vi "dialog edit search paths.vi"(8 "error in":errorcluster, 11 "Plugin Search Paths":path[](array[path])) -> (0 "error out":errorcluster, 2 "Cancelled?":bool, 3 "Plugin Search Paths":path[](array[path]))   [LabVIEW 2013, in "configuration library.lvlib"]
uses:
  configuration library.lvlib
panel:
  in  "add":bool
  in  "remove":bool
  in  "Search Paths":i32(listbox)
  in  "Cancel":bool
  in  "OK":bool
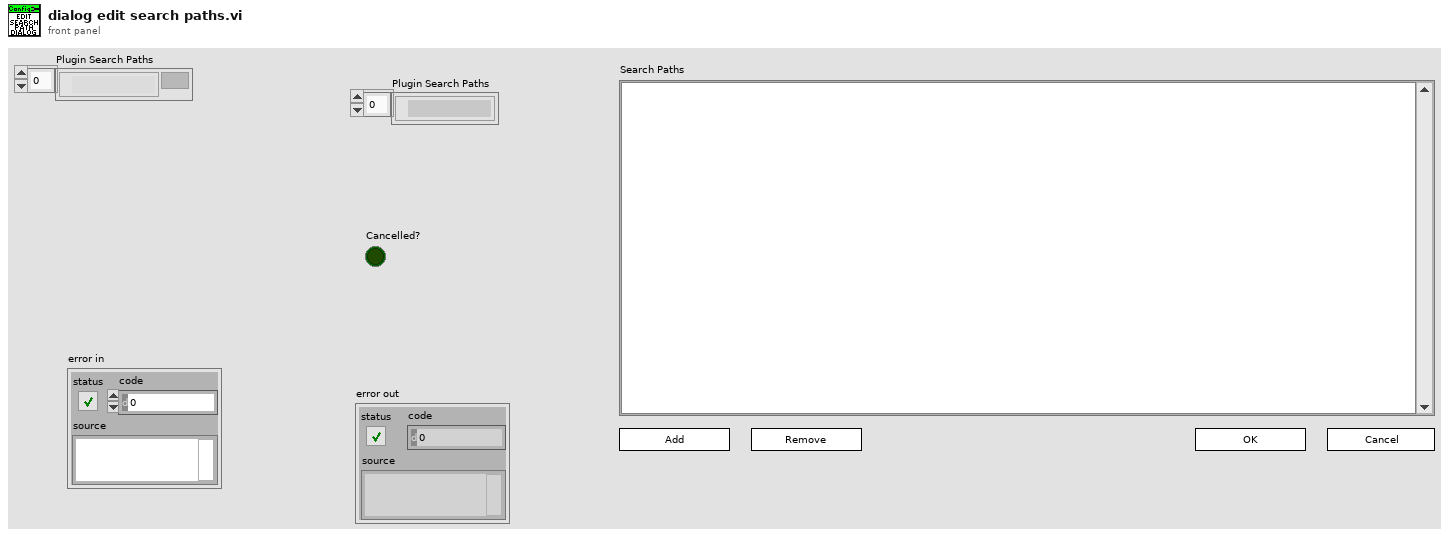
[diagram p1: front panel]
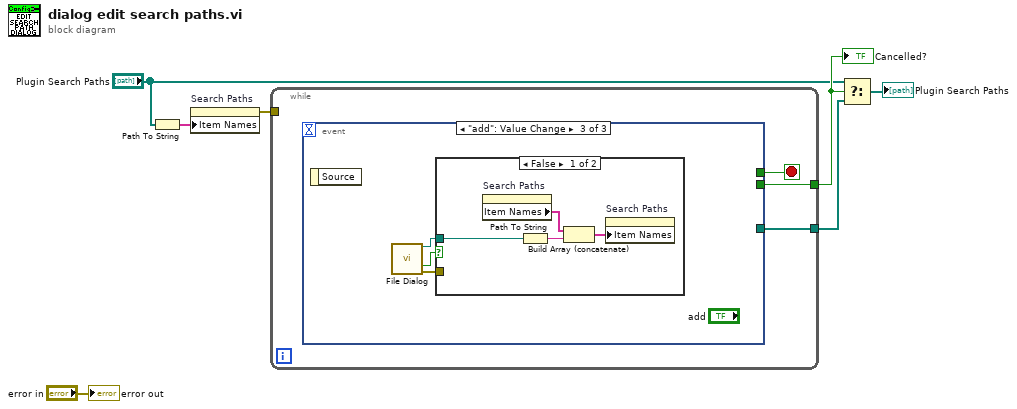
[diagram p0: block diagram]
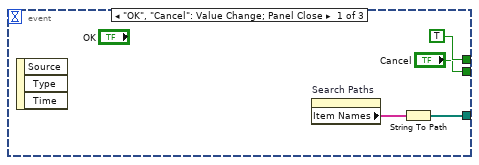
[diagram p2: hidden frame]
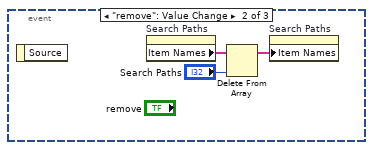
[diagram p3: hidden frame]
diagram:
  n1 = Path To String(path="Plugin Search Paths") -> (string=w2:string[])
  n2 = property on="Search Paths" class="LstBox (strict)"("Item Names"=w2) -> (error out=w1:errorcluster)  [unwired: 2 in, 1 out]
  n3 = while {
    tunnel: [w9] -> w5
    tunnel: [w8] -> w6
    tunnel: w1 -> [_]
    stop <- w10 stop-if-true
    n4 = event shown="[2] \"add\": Value Change" {
      selector: _ -> [_ _ _]
      dyn-events: _ -> [_ _ _]
      timeout: _ -> [_ _ _]
      tunnel: [TRUE _ _] -> w10
      tunnel: ["Cancel" _ _] -> w9
      tunnel: [w11 _ _] -> w8
      event "OK", "Cancel": Value Change; Panel Close {
        n5 = event-data() -> ()  [unwired: 1 in, 3 out]
        n6 = property on="Search Paths" class="LstBox (strict)"() -> ("Item Names"=w12:string[])  [unwired: 2 in, 2 out]
        n7 = String To Path(string=w12) -> (path=w11:path[])
      }
      event "remove": Value Change {
        n8 = event-data() -> ()  [unwired: 1 in, 1 out]
        n9 = property on="Search Paths" class="LstBox (strict)"() -> ("Item Names"=w17:string[])  [unwired: 2 in, 2 out]
        n10 = Delete From Array(array=w17, index="Search Paths") -> (array with subset deleted=w16:string[])  [unwired: 1 in, 1 out]
        n11 = property on="Search Paths" class="LstBox (strict)"("Item Names"=w16) -> ()  [unwired: 2 in, 2 out]
      }
      event "add": Value Change {
        n12 = event-data() -> ()  [unwired: 1 in, 1 out]
        n13 = call "File Dialog"() -> ("selected path"=w18:path, "cancelled"=w20:bool, "error out"=w19:errorcluster)  [unwired: 12 in, 1 out]
        n14 = case shown="False" w20 {
          tunnel: w19 -> [_ _]
          tunnel: w18 -> [w21 _]
          frame False {
            n15 = property on="Search Paths" class="LstBox (strict)"() -> ("Item Names"=w22:string[])  [unwired: 2 in, 2 out]
            n16 = Path To String(path=w21) -> (string=w24:string)
            n17 = Build Array (concatenate)(w22, w24) -> (w23:string[])
            n18 = property on="Search Paths" class="LstBox (strict)"("Item Names"=w23) -> ()  [unwired: 2 in, 2 out]
          }
          frame True {
          }
        }
      }
    }
  }
  "Cancelled?" <- w5
  n19 = Select(t="Plugin Search Paths", s=w5, f=w6) -> (s? t:f=→"Plugin Search Paths":path[])
  "error out" <- "error in"
